vi "sub_pf_cal-input.vi"(10 "yaw_rate":dbl=0.1, 11 "v":dbl=1.0) -> (3 "u":T1=[[1.0], [0.1]])   [LabVIEW 2019]
uses:
  <vilib>/Analysis/Matrix/Datatypes/RealMatrix.ctl
  <vilib>/Analysis/Matrix/NI_Matrix.lvlib
panel:
  out "열의 개수":i32=1
  out "행의 개수":i32=2
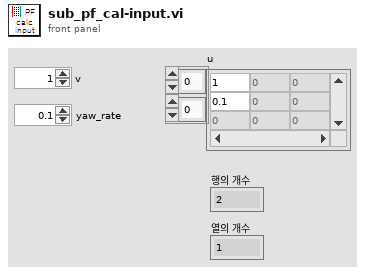
[diagram p1: front panel]
types:
  T1 = typedef "NI_Matrix.lvlib/RealMatrix.ctl" = dbl[][]
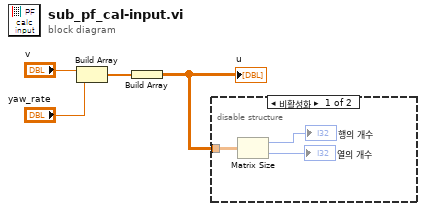
[diagram p0: block diagram]
diagram:
  n1 = Build Array("v", "yaw_rate") -> (w1:dbl[])
  n2 = Build Array(w1) -> (w2:T1)
  "u" <- w2
  n3 = disable-structure shown="비활성화" {
    disable-tunnel: w2 -> [w7 _]
    frame Disabled {
      n4 = Matrix Size(0:w7) -> (1:→"행의 개수":i32, 2:→"열의 개수":i32)
    }
    frame Enabled {
    }
  }
